vi "Check Special Tags.vi"(0 "source":string caption="Quelle") -> (1 "Before Tag (source)":string caption="Before Tag (Quelle)", 2 "After Tag (special data)":string caption="After Tag (spezielle Daten)", 3 "Tag Found?":T1 caption="Tag gefunden?")   [LabVIEW 2009]
uses:
  TagReturnType.ctl
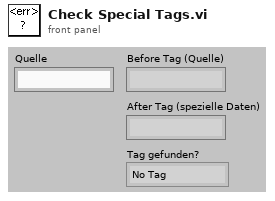
[diagram p1: front panel]
types:
  T1 = typedef "TagReturnType.ctl" = enum16{"No Tag", "<err>", "<append>"}
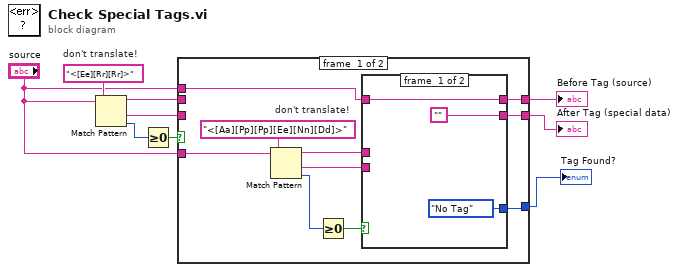
[diagram p0: block diagram]
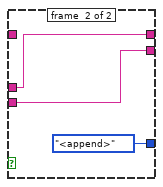
[diagram p2: hidden frame]
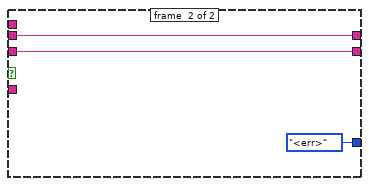
[diagram p3: hidden frame]
diagram:
  w8 = "<[Ee][Rr][Rr]>"  # don't translate!
  n1 = Match Pattern(string="source", regular expression=w8) -> (before substring=w6:string, after substring=w5:string, offset past match=w9:i32)  [unwired: 1 in, 1 out]
  n2 = Greater Or Equal To 0?(x=w9) -> (x >= 0?=w7:bool)
  n3 = case shown="False" w7 {
    tunnel: "source" -> [w17 _]
    tunnel: w6 -> [_ w27]
    tunnel: w5 -> [_ w28]
    tunnel: [w14 w28] -> w4
    tunnel: [w12 w27] -> w3
    tunnel: [w11 TagReturnType."<err>" ("Tag Found?")] -> w2
    tunnel: "source" -> [w10 _]
    frame #0 {
      w19 = "<[Aa][Pp][Pp][Ee][Nn][Dd]>"  # don't translate!
      n4 = Match Pattern(string=w17, regular expression=w19) -> (before substring=w15:string, after substring=w13:string, offset past match=w18:i32)  [unwired: 1 in, 1 out]
      n5 = Greater Or Equal To 0?(x=w18) -> (x >= 0?=w16:bool)
      n6 = case shown="False" w16 {
        tunnel: w15 -> [_ w24]
        tunnel: ["" w25] -> w14
        tunnel: w13 -> [_ w25]
        tunnel: [w20 w24] -> w12
        tunnel: [TagReturnType."No Tag" ("Tag Found?") TagReturnType."<append>" ("Tag Found?")] -> w11
        tunnel: w10 -> [w20 _]
        frame #0 {
        }
        frame #1 {
        }
      }
    }
    frame #1 {
    }
  }
  "After Tag (special data)" <- w4
  "Before Tag (source)" <- w3
  "Tag Found?" <- w2
